vi "CC Read Channels from TDMS File.vi"(8 "error in (no error)":errorcluster, 10 "Sources":string[](array[string]), 11 "ItemNames":string[](array[string])) -> (0 "error out":errorcluster, 1 "units":string[](array[string]), 2 "Y Axes":i32[](array[numeric]), 3 "XY Graph":cluster{timestamp[], dbl[]}[](graph))   [LabVIEW 2024]
uses:
  CC enum Current Values Action.ctl
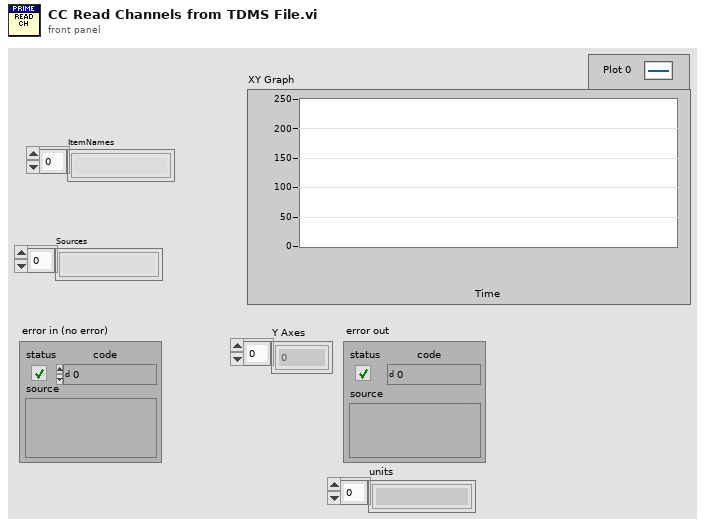
[diagram p1: front panel]
types:
  T1 = enum16{"open", "open or create", "create or replace", "create", "open (read-only)"}
  T2 = typedef "CC enum Current Values Action.ctl" = enum16{"Init", "Write Item", "Write Array", "Read Item", "Read Array", "Read All", "Add Channels", "New File", "Add Message", "Get Current Values", "Close"}
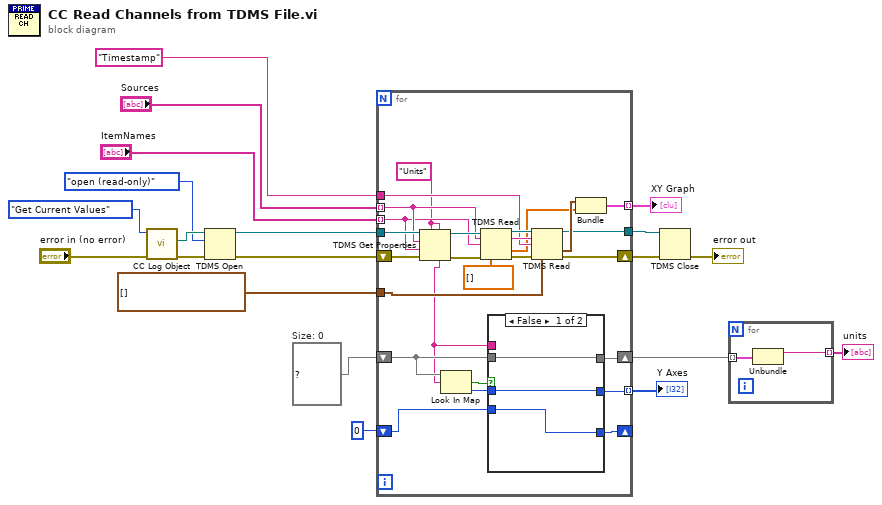
[diagram p0: block diagram]
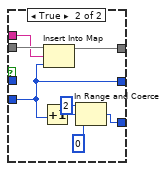
[diagram p2: hidden frame]
diagram:
  w5 = map{string, i32} {}  # Size: 0
  n1 = call "CC Log Object.vi"("error in (no error)"="error in (no error)", "Action"=CC_enum_Current_Values_Action."Get Current Values") -> ("error out"=w10:errorcluster, "Current File"=w19:path)  [unwired: 7 in, 1 out]
  n2 = TDMS Open(8:w10, 10:T1."open (read-only)" ("operation (0:open)"), 11:w19) -> (0:w11:errorcluster, 3:w17:refnum<k34>)  [unwired: 4 in]
  n3 = for {
    tunnel: w17 -> [w32]
    tunnel: "Timestamp" -> [w43]
    tunnel: timestamp[] [] -> [w42]
    tunnel: [w38] -> w14 mode=indexing
    tunnel: [w37] -> w13
    shift-right: [w36] -> w12
    shift-left: w11 -> [w33]
    tunnel: "Sources" -> [w31] mode=indexing
    tunnel: "ItemNames" -> [w30] mode=indexing
    shift-right: [w24] -> w3
    shift-left: w5 -> [w25]
    shift-right: [w22] -> _
    shift-left: 0 -> [w26]
    tunnel: [w21] -> w1 mode=indexing
    w29 = "Units" ("property name")
    n4 = TDMS Get Properties(5:w29, 7:w29, 8:w33, 9:w30, 10:w31, 11:w32) -> (0:w35:errorcluster, 3:w34:refnum<k34>, 4:w23:string)  [unwired: 3 out]
    n5 = Look In Map(map=w25, key=w23) -> (key not found?=w28:bool, value=w27:i32)  [unwired: 1 in]
    n6 = TDMS Read(0:w34, 5:w31, 7:w30, 11:w35, 12:dbl[] []) -> (4:w45:refnum<k34>, 6:w44:string, 10:w39:dbl[], 15:w41:errorcluster)  [unwired: 3 in, 2 out]
    n7 = case shown="False" w28 {
      tunnel: w27 -> [w47 _]
      tunnel: w26 -> [w48 w50]
      tunnel: w25 -> [w49 w57]
      tunnel: [w49 w56] -> w24
      tunnel: w23 -> [_ w55]
      tunnel: [w48 w51] -> w22
      tunnel: [w47 w50] -> w21
      frame False {
      }
      frame True {
        n8 = Increment(x=w50) -> (x+1=w54:i32)
        n9 = Insert Into Map(map in=w57, key=w55, value=w50) -> (map out=w56:map{string, i32})  [unwired: 2 out]
        n10 = In Range and Coerce(upper limit=2, x=w54, lower limit=0) -> (coerced(x)=w51:i32)  [unwired: 1 out]
      }
    }
    n11 = TDMS Read(0:w45, 5:w44, 7:w43, 11:w41, 12:w42) -> (4:w37:refnum<k34>, 10:w40:timestamp[], 15:w36:errorcluster)  [unwired: 3 in, 3 out]
    n12 = Bundle(w40, w39) -> (w38:cluster{timestamp[], dbl[]})  [unwired: 1 in]
  }
  "XY Graph" <- w14
  "Y Axes" <- w1
  n13 = TDMS Close(8:w12, 11:w13) -> (0:→"error out":errorcluster)  [unwired: 1 out]
  n14 = for {
    tunnel: w3 -> [w59] mode=indexing
    tunnel: [w58] -> w2 mode=indexing
    n15 = Unbundle(w59) -> (w58:string)  [unwired: 1 out]
  }
  "units" <- w2
